vi "Read Worker Type.vi"(8 "error in (no error)":errorcluster, 11 "Cashier in":refnum<class "Cashier.lvclass">) -> (0 "error out":errorcluster, 2 "Type":string, 3 "Cashier out":refnum<class "Cashier.lvclass">)   [LabVIEW 2023, in "Cashier.lvclass"]
doc: "Returns the type of worker. This method is required by any descendant of the Worker class.\n\nBecause this method is implemented by the Cashier class, it will always return \"Cashier.\""
uses:
  Cashier.lvclass
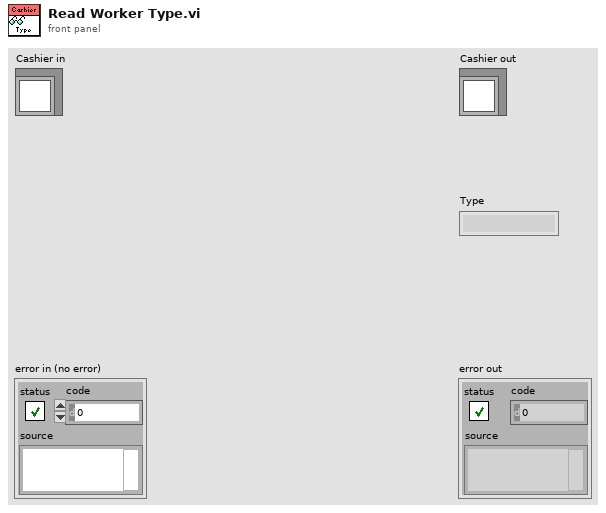
[diagram p1: front panel]
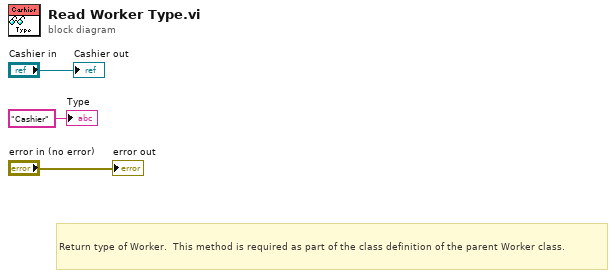
[diagram p0: block diagram]
diagram:
  # "Return type of Worker.  This method is required as part of the class definition of the parent Worker class."
  "error out" <- "error in (no error)"
  "Cashier out" <- "Cashier in"
  "Type" <- "Cashier" ("Type")
